vi "Set Color by ColorBox.vi"(8 "error in (no error)":errorcluster caption="错误输入（无错误）", 11 "Colorbox":u32(colorbox)) -> (0 "error out":errorcluster caption="错误输出", 3 "FromArgb":refnum<k24>)   [LabVIEW 2012, in "Color.lvclass"]
uses:
  Color.lvclass
  System.Drawing
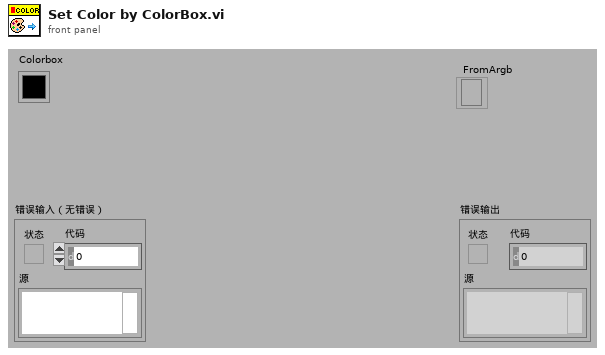
[diagram p1: front panel]
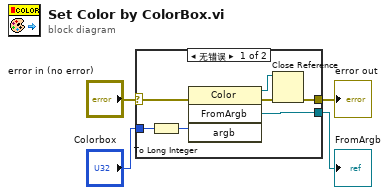
[diagram p0: block diagram]
diagram:
  n1 = case shown="无错误" "error in (no error)" {
    selector: "error in (no error)" -> [w9 w12]
    tunnel: [w8 w12] -> w3
    tunnel: "Colorbox" -> [w11 _]
    tunnel: [w5 _] -> w1
    frame No Error {
      n2 = To Long Integer(number=w11) -> (32bit integer=w10:i32)
      n3 = invoke class="Color" method="FromArgb"(error in=w9, "argb"=w10) -> (reference out=w7:refnum<k24>, error out=w6:errorcluster, "FromArgb"=w5:refnum<k24>)  [unwired: 2 in, 1 out]
      n4 = Close Reference(reference=w7, error in (no error)=w6) -> (error out=w8:errorcluster)
    }
    frame Error {
    }
  }
  "error out" <- w3
  "FromArgb" <- w1
